vi "close.vi"(8 "error in":errorcluster, 11 "CVT runtime in":refnum<class "CVT runtime.lvclass">) -> (0 "error out":errorcluster)   [LabVIEW 2013, in "CVT runtime.lvclass"]
doc: "Provides an interface for terminating a module instance. While this interface performs no operations, a child should close and deallocate any open references or memory."
uses:
  CVT runtime.lvclass
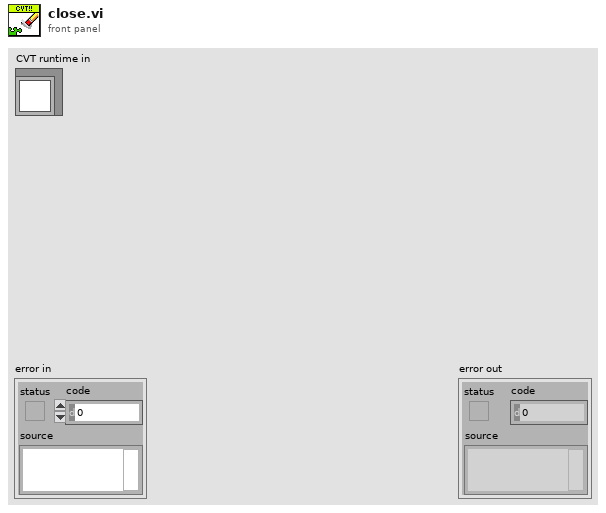
[diagram p1: front panel]
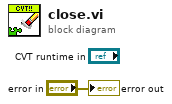
[diagram p0: block diagram]
diagram:
  "error out" <- "error in"
